vi "Write time.vi"(8 "error in (no error)":errorcluster, 10 "time":timestamp, 11 "CRDS Data in":refnum<class "CRDS Data.lvclass">=refnum) -> (0 "error out":errorcluster, 3 "CRDS Data out":refnum<class "CRDS Data.lvclass">)   [LabVIEW 2012, in "CRDS Data.lvclass"]
uses:
  CRDS Data.lvclass
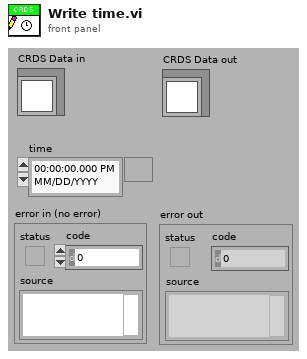
[diagram p1: front panel]
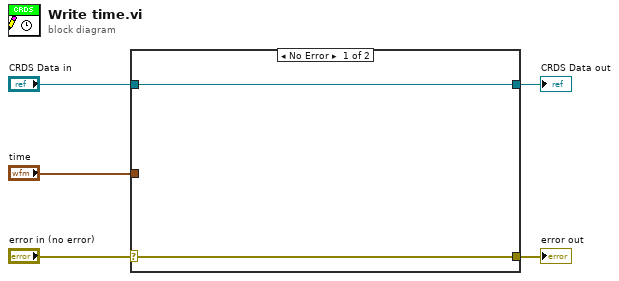
[diagram p0: block diagram]
diagram:
  n1 = case shown="No Error" "error in (no error)" {
    selector: "error in (no error)" -> [w7 w8]
    tunnel: [w7 w8] -> w4
    tunnel: [w6 w9] -> w2
    tunnel: "CRDS Data in" -> [w6 w9]
    tunnel: "time" -> [_ _]
    frame No Error {
    }
    frame Error {
    }
  }
  "error out" <- w4
  "CRDS Data out" <- w2
